vi "Self-consistent charge neutrality.vi"(4 "Volume (A³)":dbl=7795.605843681768, 6 "Chemical Potential (0=Cd, 1=Te)":dbl(slide) scale=0.0..1.0, 8 "CBM (eV)":dbl=3.2, 9 "VBM (eV)":dbl=1.79581, 10 "Temperature (K)":dbl(slide)=300.0 scale=77.0..800.0, 11 "Defects":T1(array[cluster])) -> (3 "Thermodynamic Fermi Level (eV) - VBM":dbl)   [LabVIEW 2010]
panel:
  in  "Dielectric Constant":dbl=11.0
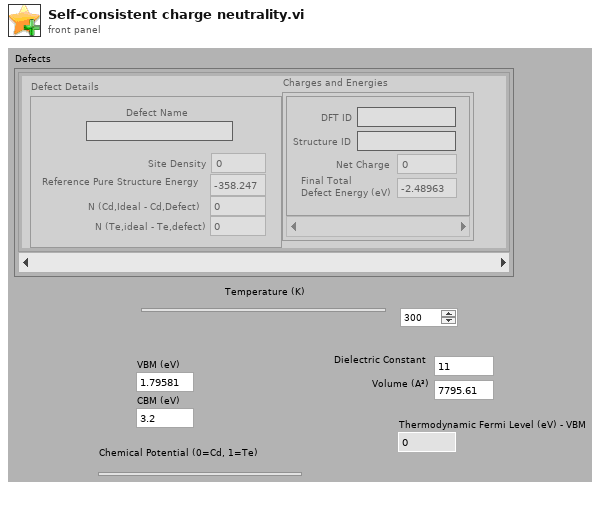
[diagram p1: front panel]
types:
  T1 = cluster{"Defect Details":cluster{"Defect Name":string, "Site Density":dbl, "Reference Pure Structure Energy":dbl, "N (Cd,Ideal - Cd,Defect)":i32, "N (Te,ideal - Te,defect)":i32}, "Charges and Energies":cluster{"DFT ID":string, "Structure ID":string, "Net Charge":i32, "Final Total \nDefect Energy (eV)":dbl}[]}[]
  T2 = cluster{"Defect Name":string, "Site Density":dbl, "Reference Pure Structure Energy":dbl, "N (Cd,Ideal - Cd,Defect)":i32, "N (Te,ideal - Te,defect)":i32}
  T3 = cluster{"DFT ID":string, "Structure ID":string, "Net Charge":i32, "Final Total \nDefect Energy (eV)":dbl}[]
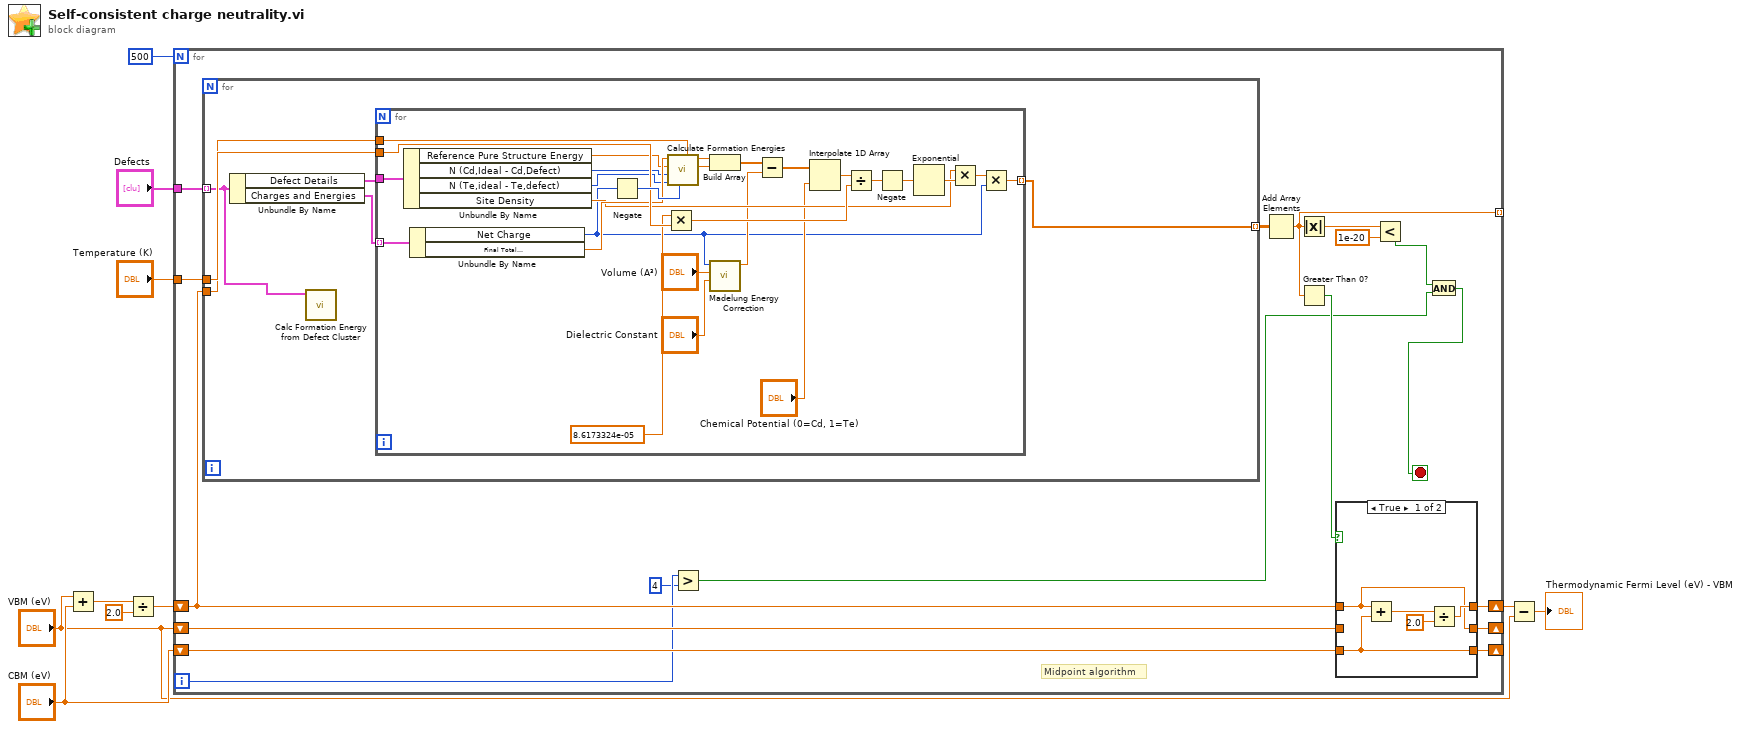
[diagram p0: block diagram]
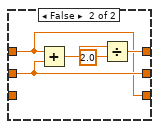
[diagram p2: hidden frame]
diagram:
  n1 = Add(x="VBM (eV)", y="CBM (eV)") -> (x+y=w10:dbl)
  n2 = Divide(x=w10, y=2.0) -> (x/y=w7:dbl)
  n3 = for {
    N: 500 -> [_]
    shift-right: [w22] -> w2
    shift-left: w7 -> [w17]
    tunnel: "Temperature (K)" -> [w28]
    tunnel: [w24] -> _ mode=indexing
    shift-right: [w19] -> _
    shift-left: "VBM (eV)" -> [w20]
    shift-right: [w18] -> _
    shift-left: "CBM (eV)" -> [w21]
    tunnel: "Defects" -> [w16]
    i -> [w12]
    stop <- w13 stop-if-true
    # "Midpoint algorithm"
    n4 = for {
      tunnel: w17 -> [w42]
      tunnel: w28 -> [w44]
      tunnel: [w43] -> w27 mode=indexing
      tunnel: w16 -> [w39] mode=indexing
      n5 = Unbundle By Name(w39) -> ("Defect Details"=w40:T2, "Charges and Energies"=w41:T3)
      n6 = call "Calc Formation Energy from Defect Cluster.vi"("Defect Data"=w39) -> ()  [unwired: 9 in, 2 out]
      n7 = for {
        tunnel: w44 -> [w67]
        tunnel: [w63] -> w43 mode=indexing
        tunnel: w42 -> [w62]
        tunnel: w41 -> [w60] mode=indexing
        tunnel: w40 -> [w61]
        n8 = Unbundle By Name(w61) -> ("Reference Pure Structure Energy"=w58:dbl, "N (Cd,Ideal - Cd,Defect)"=w57:i32, "N (Te,ideal - Te,defect)"=w56:i32, "Site Density"=w55:dbl)
        n9 = Unbundle By Name(w60) -> ("Net Charge"=w48:i32, "Final Total \nDefect Energy (eV)"=w59:dbl)
        n10 = Negate(x=w48) -> (-x=w71:i32)
        n11 = Multiply(x=8.6173324e-05, y=w67) -> (x*y=w68:dbl)
        n12 = call "Calculate Formation Energies.vi"("Fermi (electron) energy (eV)"=w62, "# Extra Electrons"=w71, "N (Te,ideal - Te,defect)"=w56, "N (Cd,Ideal - Cd,Defect)"=w57, "Reference Pure Structure Energy"=w58, "Final Total Defect Energy (eV)"=w59) -> ("Formation Energy (Te-Rich)"=w53:dbl, "Formation Energy (Cd-Rich)"=w54:dbl)  [unwired: 4 in]
        n13 = Build Array(w54, w53) -> (w50:dbl[])
        n14 = call "Madelung Energy Correction.vi"("Dielectric Constant"="Dielectric Constant", "Volume (A³)"="Volume (A³)", "Net Charge"=w48) -> ("1st Order correction (eV)"=w49:dbl)  [unwired: 7 in, 1 out]
        n15 = Subtract(x=w50, y=w49) -> (x-y=w45:dbl[])
        n16 = Interpolate 1D Array(1:"Chemical Potential (0=Cd, 1=Te)", 2:w45) -> (0:w51:dbl)
        n17 = Divide(x=w51, y=w68) -> (x/y=w70:dbl)
        n18 = Negate(x=w70) -> (-x=w69:dbl)
        n19 = Exponential(1:w69) -> (0:w65:dbl)
        n20 = Multiply(x=w55, y=w65) -> (x*y=w64:dbl)
        n21 = Multiply(x=w64, y=w48) -> (x*y=w63:dbl)
      }
    }
    n22 = Greater?(x=w12, y=4) -> (0:w14:bool)
    n23 = Add Array Elements(numeric array=w27) -> (sum=w24:dbl)
    n24 = Absolute Value(x=w24) -> (abs(x)=w26:dbl)
    n25 = Greater Than 0?(x=w24) -> (x > 0?=w23:bool)
    n26 = case shown="True" w23 {
      tunnel: w17 -> [w30 w34]
      tunnel: [w31 w36] -> w22
      tunnel: w21 -> [w29 _]
      tunnel: w20 -> [_ w35]
      tunnel: [w30 w35] -> w19
      tunnel: [w29 w34] -> w18
      frame True {
        n27 = Add(x=w30, y=w29) -> (x+y=w33:dbl)
        n28 = Divide(x=w33, y=2.0) -> (x/y=w31:dbl)
      }
      frame False {
        n29 = Add(x=w34, y=w35) -> (x+y=w38:dbl)
        n30 = Divide(x=w38, y=2.0) -> (x/y=w36:dbl)
      }
    }
    n31 = Less?(x=w26, y=1e-20) -> (x < y?=w15:bool)
    n32 = And(x=w15, y=w14) -> (x .and. y?=w13:bool)
  }
  n33 = Subtract(x=w2, y="VBM (eV)") -> (x-y=→"Thermodynamic Fermi Level (eV) - VBM":dbl)
